vi "test_libssh2_session_init_ex (send callback).vi"() -> ()   [LabVIEW 2013, in "libssh2_integration_tests.lvlib"]
uses:
  libssh2_integration_tests.lvlib
  libssh2/libssh2_session_abstract.ctl
  libssh2/libssh2_session_callback_type.ctl
  Server Fixture/Server Fixture.lvclass/Server Fixture.ctl
  Server Fixture/Read User Private Key File.vi
  Server Fixture/Read User Public Key File.vi
  Server Fixture/Read User Name.vi
  Server Fixture/Read User Private Key Passphrase.vi
  Server Fixture/Read Server Address.vi
  Server Fixture/Read Server Port.vi
  callback_send.vi
  libssh2/libssh2_init_default.vi
  libssh2/libssh2_session_handshake_tcp.vi
  libssh2/libssh2.lvlib
  Server Fixture/Server Fixture.lvclass
  <vilib>/addons/_JKI Toolkits/Caraya/classes/Assert/Assert.lvclass
  <vilib>/addons/_JKI Toolkits/Caraya/classes/Test/Test.lvclass
panel:
  out "error out":errorcluster
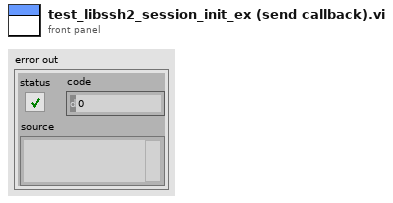
[diagram p1: front panel]
types:
  T1 = typedef "libssh2.lvlib/libssh2_session_callback_type.ctl" = enum16{"Ignore", "Debug", "Disconnect", "MAC Error", "X11", "Send", "Receive", "Auth Agent", "Auth Agent Identities", "Auth Agent Sign"}
  T2 = typedef "libssh2.lvlib/libssh2_session_abstract.ctl" = cluster{"send":refnum<vi>, "receive":refnum<vi>}
  T3 = typedef "libssh2.lvlib/Session Refnum.ctl" = refnum<k1>
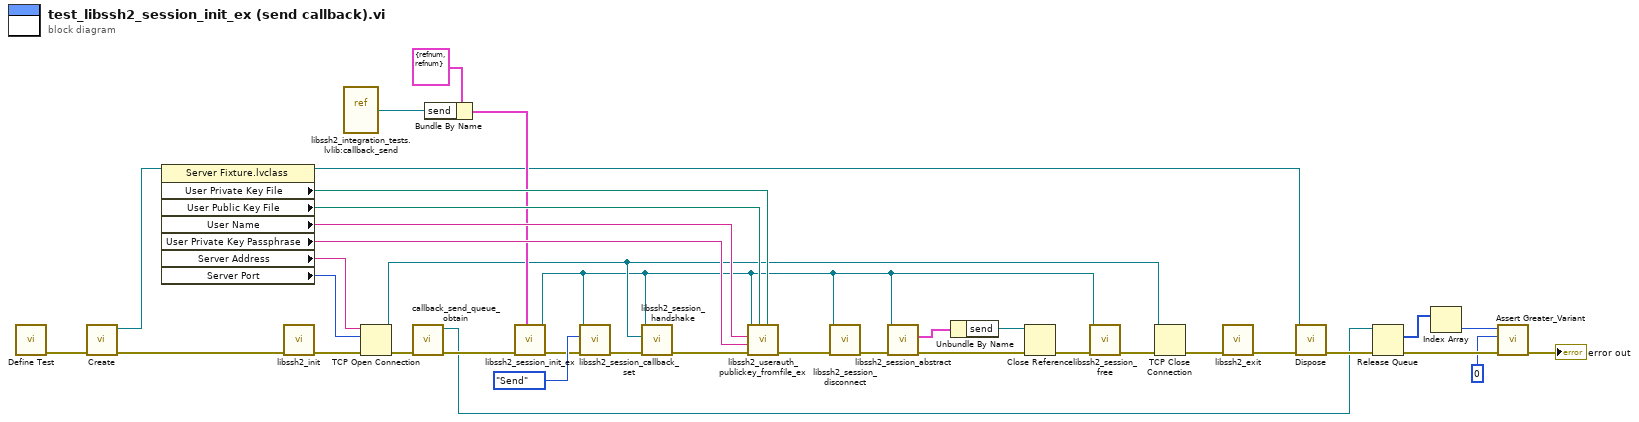
[diagram p0: block diagram]
diagram:
  n1 = call <vilib>:"Define Test.vi"() -> ("error out"=w7:errorcluster)  [unwired: 10 in, 1 out]
  n2 = call "Create.vi"("error in (no error)"=w7) -> ("error out"=w32:errorcluster, "Server Fixture"=w31:refnum<class "Server Fixture.lvclass">)  [unwired: 9 in]
  n3 = property on="Property Node" class="Server Fixture.lvclass"(reference=w31) -> (reference out=w18:refnum<class "Server Fixture.lvclass">, "User Private Key File"=w36:path, "User Public Key File"=w37:path, "User Name"=w35:string, "User Private Key Passphrase"=w34:string, "Server Address"=w30:string, "Server Port"=w29:u16)  [unwired: 1 in, 1 out]
  n4 = call-poly "libssh2_init.vi"("error in (no error)"=w32) -> ("error out"=w38:errorcluster)  [unwired: 10 in]
  n5 = vi-ref "libssh2_integration_tests.lvlib:callback_send.vi"() -> (w26:refnum<vi>)
  n6 = TCP Open Connection(address=w30, remote port or service name=w29, error in (no error)=w38) -> (connection ID=w19:refnum<k5>, error out=w14:errorcluster)  [unwired: 2 in]
  n7 = call "callback_send_queue_obtain.vi"("error in (no error)"=w14) -> ("error out"=w13:errorcluster, "queue out"=w11:refnum<queue>)  [unwired: 9 in]
  n8 = Bundle By Name(cluster=T2 {"send"=refnum, "receive"=refnum} ("abstract"), "send"=w26) -> (w27:T2)
  n9 = call "libssh2_session_init_ex.vi"("abstract"=w27, "error in (no error)"=w13) -> ("error out"=w24:errorcluster, "session"=w17:T3)  [unwired: 8 in]
  n10 = call "libssh2_session_callback_set.vi"("error in (no error)"=w24, "callback type"=libssh2_session_callback_type."Send", "session"=w17) -> ("error out"=w9:errorcluster)  [unwired: 7 in, 1 out]
  n11 = call-poly "libssh2_session_handshake.vi"("error in (no error)"=w9, "tcp connection"=w19, "session"=w17) -> ("error out"=w33:errorcluster)  [unwired: 8 in]
  n12 = call "libssh2_userauth_publickey_fromfile_ex.vi"("private key"=w36, "public key"=w37, "error in (no error)"=w33, "passphrase"=w34, "username"=w35, "session"=w17) -> ("error out"=w2:errorcluster)  [unwired: 5 in]
  n13 = call "libssh2_session_disconnect.vi"("error in (no error)"=w2, "session"=w17) -> ("error out"=w3:errorcluster)  [unwired: 9 in]
  n14 = call "libssh2_session_abstract.vi"("error in (no error)"=w3, "session"=w17) -> ("error out"=w8:errorcluster, "abstract"=w15:T2)  [unwired: 8 in]
  n15 = Unbundle By Name(w15) -> ("send"=w16:refnum<vi>)
  n16 = Close Reference(reference=w16, error in (no error)=w8) -> (error out=w4:errorcluster)
  n17 = call "libssh2_session_free.vi"("error in (no error)"=w4, "session"=w17) -> ("error out"=w23:errorcluster)  [unwired: 9 in]
  n18 = TCP Close Connection(connection ID=w19, error in (no error)=w23) -> (error out=w22:errorcluster)  [unwired: 1 in, 1 out]
  n19 = call "libssh2_exit.vi"("error in (no error)"=w22) -> ("error out"=w21:errorcluster)  [unwired: 10 in]
  n20 = call "Dispose.vi"("error in (no error)"=w21, "Server Fixture in"=w18) -> ("error out"=w20:errorcluster)  [unwired: 7 in, 2 out]
  n21 = Release Queue(queue=w11, error in (no error)=w20) -> (remaining elements=w6:i64[], error out=w12:errorcluster)  [unwired: 1 in, 1 out]
  n22 = Index Array(array=w6) -> (element=w1:i64)  [unwired: 1 in]
  n23 = call <vilib>:"Assert Greater_Variant.vi"("error in (no error)"=w12, "Y"=i64 0, "X"=w1) -> ("error out"=→"error out":errorcluster)  [unwired: 7 in, 1 out]
